vi "test_tx-rx-loopback.vi"(0 "USRP IP address":string="192.168.10.88", 1 "RFNoC Graph Settings":T2, 2 "Tx Settings":T1={"frequency"=2000000000.0, "rate"=1000000.0, "antenna"="TX/RX0", "gain"=0.0}, 3 "Rx Settings":T1={"frequency"=2000000000.0, "rate"=1000000.0, "antenna"="RX1", "gain"=0.0}, 5 "Iteration Count":u32=10000, 7 "Python Version":string(combo)="3.10", 11 "error in (no error)":errorcluster) -> (4 "Pass":bool, 6 "Results":string, 15 "error out":errorcluster)   [LabVIEW 2024]
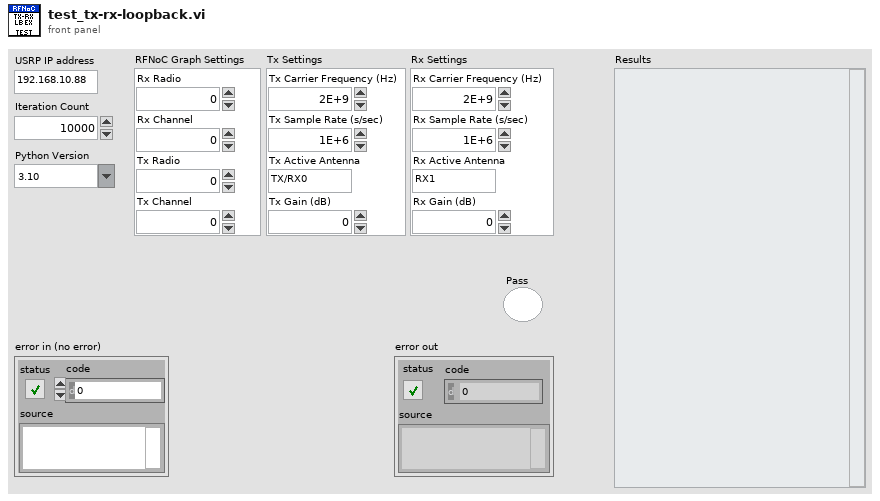
[diagram p1: front panel]
types:
  T1 = cluster{"frequency":dbl, "rate":dbl, "antenna":string, "gain":dbl}
  T2 = cluster{"rx_radio":u32, "rx_chan":u32, "tx_radio":u32, "tx_chan":u32}
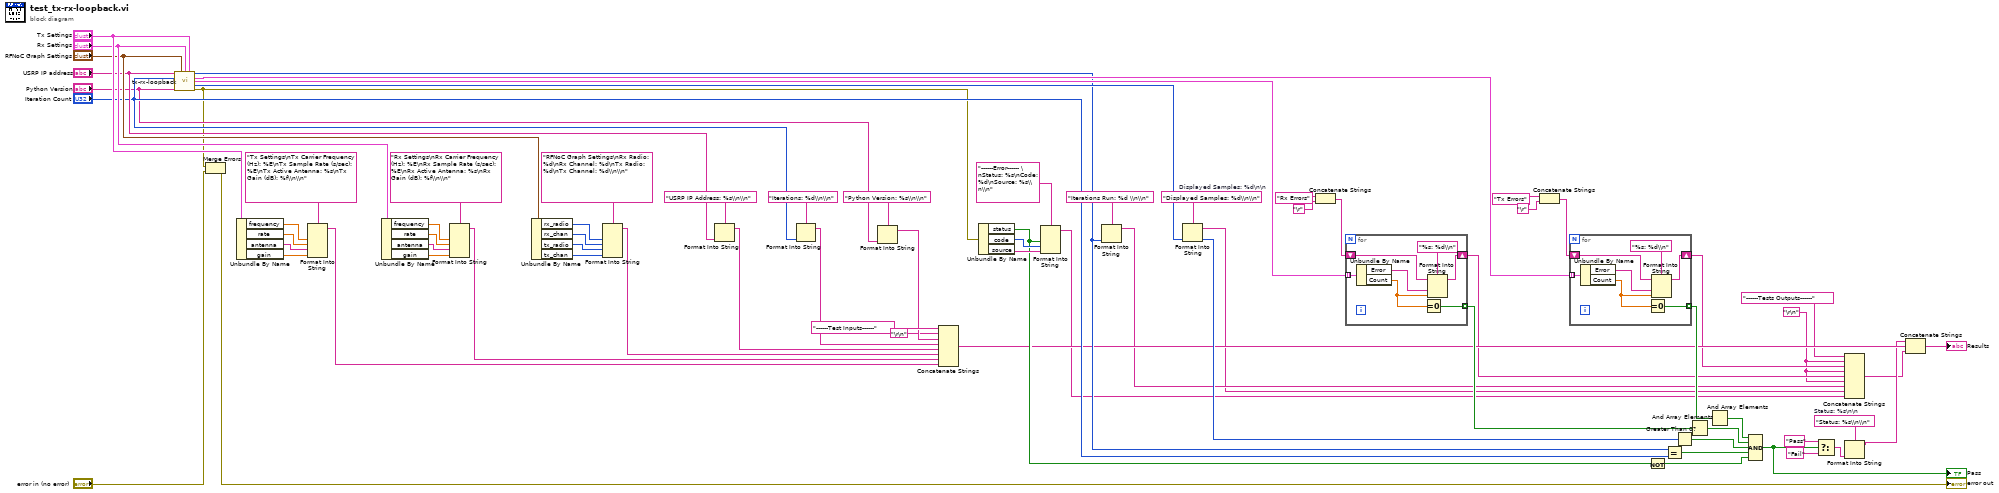
[diagram p0: block diagram]
diagram:
  w11 = "\r\n"
  w64 = "Displayed Samples: %d\\n\\n"  # Displayed Samples: %d\n\n
  w55 = "Status: %s\\n\\n"  # Status: %s\n\n
  n1 = call "tx-rx-loopback.vi"("USRP IP address"="USRP IP address", "RFNoC Graph Settings"="RFNoC Graph Settings", "Rx Settings"="Rx Settings", "Tx Settings"="Tx Settings", "Iteration Count"="Iteration Count", "Python Version"="Python Version") -> ("Iterations"=w62:u32, "Tx Errors"=w74:cluster{"Error":string, "Count":dbl}[], "Rx Errors"=w67:cluster{"Error":string, "Count":dbl}[], "Displayed Samples"=w63:u64, "Error"=w2:errorcluster)  [unwired: 5 in]
  n2 = Merge Errors(w2, "error in (no error)") -> (→"error out":errorcluster)
  n3 = Unbundle By Name("Tx Settings") -> ("frequency"=w53:dbl, "rate"=w52:dbl, "antenna"=w51:string, "gain"=w50:dbl)
  n4 = Format Into String(format string="Tx Settings\nTx Carrier Frequency (Hz): %E\nTx Sample Rate (s/sec): %E\nTx Active Antenna: %s\nTx Gain (dB): %f\\n\\n", w53, w52, w51, w50) -> (resulting string=w20:string)  [unwired: 2 in, 1 out]
  n5 = Unbundle By Name("Rx Settings") -> ("frequency"=w43:dbl, "rate"=w44:dbl, "antenna"=w45:string, "gain"=w46:dbl)
  n6 = Format Into String(format string="Rx Settings\nRx Carrier Frequency (Hz): %E\nRx Sample Rate (s/sec): %E\nRx Active Antenna: %s\nRx Gain (dB): %f\\n\\n", w43, w44, w45, w46) -> (resulting string=w21:string)  [unwired: 2 in, 1 out]
  n7 = Unbundle By Name("RFNoC Graph Settings") -> ("rx_radio"=w41:u32, "rx_chan"=w40:u32, "tx_radio"=w39:u32, "tx_chan"=w38:u32)
  n8 = Format Into String(format string="RFNoC Graph Settings\nRx Radio: %d\nRx Channel: %d\nTx Radio: %d\nTx Channel: %d\\n\\n", w41, w40, w39, w38) -> (resulting string=w22:string)  [unwired: 2 in, 1 out]
  n9 = Format Into String(format string="USRP IP Address: %s\\n\\n", "USRP IP address") -> (resulting string=w23:string)  [unwired: 2 in, 1 out]
  n10 = Format Into String(format string="Iterations: %d\\n\\n", "Iteration Count") -> (resulting string=w24:string)  [unwired: 2 in, 1 out]
  n11 = Format Into String(format string="Python Version: %s\\n\\n", "Python Version") -> (resulting string=w25:string)  [unwired: 2 in, 1 out]
  n12 = Concatenate Strings("------Test Inputs------" ("string"), "\r\n", w25, w24, w23, w22, w21, w20) -> (w15:string)
  n13 = Unbundle By Name(w2) -> ("status"=w16:bool, "code"=w18:i32, "source"=w17:string)
  n14 = Format Into String(format string="------Error------ \nStatus: %s\nCode: %d\nSource: %s\\n\\n", w16, w18, w17) -> (resulting string=w5:string)  [unwired: 2 in, 1 out]
  n15 = Format Into String(format string="Iterations Run: %d \\n\\n" ("initial string"), w62) -> (resulting string=w10:string)  [unwired: 2 in, 1 out]
  n16 = Format Into String(format string=w64, w63) -> (resulting string=w9:string)  [unwired: 2 in, 1 out]
  n17 = Concatenate Strings("Rx Errors", "\r") -> (w70:string)
  n18 = for {
    tunnel: w67 -> [w81] mode=indexing
    shift-right: [w78] -> w12
    shift-left: w70 -> [w77]
    tunnel: [w75] -> w65 mode=indexing
    n19 = Unbundle By Name(w81) -> ("Error"=w79:string, "Count"=w76:dbl)
    n20 = Equal To 0?(x=w76) -> (x = 0?=w75:bool)
    n21 = Format Into String(format string="%s: %d\\n", initial string=w77, w79, w76) -> (resulting string=w78:string)  [unwired: 1 in, 1 out]
  }
  n22 = Concatenate Strings("Tx Errors", "\r") -> (w71:string)
  n23 = for {
    tunnel: w74 -> [w88] mode=indexing
    shift-right: [w85] -> w13
    shift-left: w71 -> [w84]
    tunnel: [w82] -> w66 mode=indexing
    n24 = Unbundle By Name(w88) -> ("Error"=w86:string, "Count"=w83:dbl)
    n25 = Equal To 0?(x=w83) -> (x = 0?=w82:bool)
    n26 = Format Into String(format string="%s: %d\\n", initial string=w84, w86, w83) -> (resulting string=w85:string)  [unwired: 1 in, 1 out]
  }
  n27 = Not(x=w16) -> (.not. x?=w6:bool)
  n28 = Equal?(x=w62, y="Iteration Count") -> (x = y?=w60:bool)
  n29 = Greater Than 0?(x=w63) -> (x > 0?=w27:bool)
  n30 = And Array Elements(Boolean array=w65) -> (logical AND=w28:bool)
  n31 = And Array Elements(Boolean array=w66) -> (logical AND=w29:bool)
  n32 = Compound Arithmetic op=AND(w29, w28, w27, w60, w6) -> (w57:bool)
  "Pass" <- w57
  n33 = Select(t="Pass", s=w57, f="Fail") -> (s? t:f=w54:string)
  n34 = Concatenate Strings("------Tests Outputs------" ("string"), w11, w13, w11, w12, w11, w10, w9, w5) -> (w7:string)
  n35 = Format Into String(format string=w55, w54) -> (resulting string=w8:string)  [unwired: 2 in, 1 out]
  n36 = Concatenate Strings(w8, w15, w7) -> (→"Results":string)
